vi "_FPGA_DDS_BMem_of_Cosine.vi"(8 "Addr":enum16{"Addr A", "Addr B"}(ring)=enum."Addr B", 10 "Cycle_in":u32, 11 "NormAmp*2^29":u32) -> (2 "cos":fxp<+/-,16,14>)   [LabVIEW 2018]
uses:
  <vilib>/rvi/Memory/Memory_Emulation/nirvimemoryFastEmulation.vi
  <vilib>/rvi/Memory/Memory_Emulation/nirvimemoryEmulation.vi
  <vilib>/rvi/Emulation/niFpgaEmulationIsFPGAContextNoSignature.vi
  <vilib>/rvi/DataTransferAndStorage/Container/Common/niFpgaContainerGetUniqueNameForEmu.vi
  <vilib>/rvi/Emulation/niFpgaProcessEmulError.vi
  <vilib>/rvi/Emulation/niFpgaSctlEmulationGetInTimedLoop.vi
  <vilib>/rvi/errors/nirviReportUnexpectedCaseInternalError (U32).vi
  <vilib>/rvi/DataTransferAndStorage/Container/XNode/niFpgaContainer.xnode
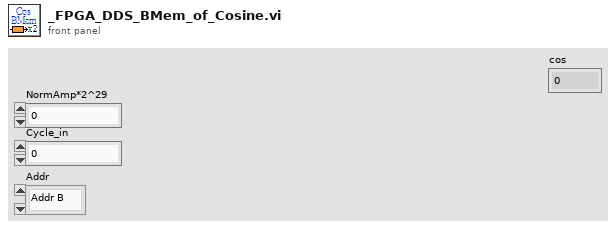
[diagram p1: front panel]
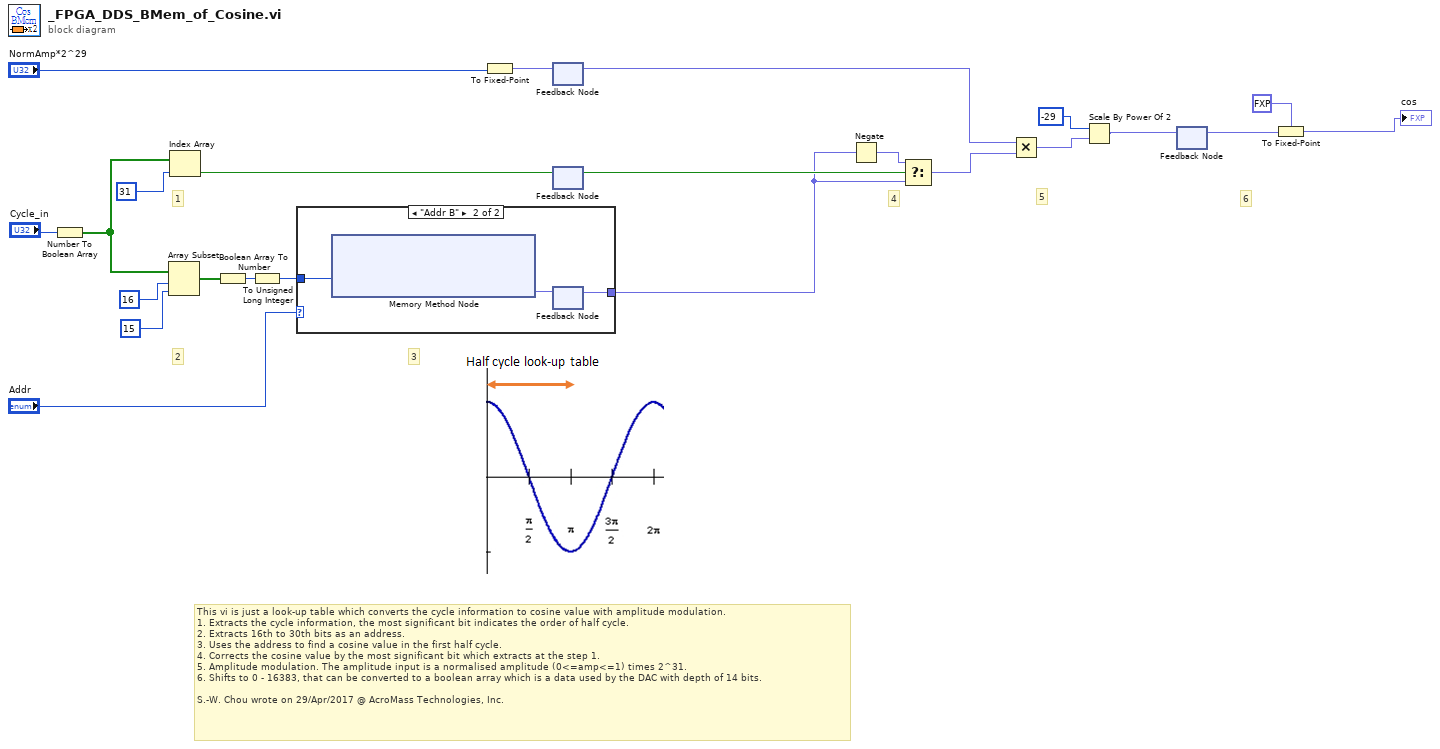
[diagram p0: block diagram]
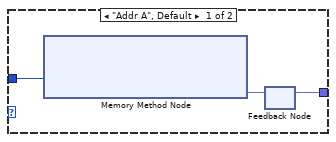
[diagram p2: hidden frame]
diagram:
  # "6"
  # "5"
  # "4"
  # "3"
  # "1"
  # "2"
  # "This vi is just a look-up table which converts the cycle information to cosine value with amplitude modulation.\n1. Extracts the cycle information, the most significant bit indicates the order of half cycle.\n2. Extracts 16th to 30th bits as an address.\n3. Uses the address to find a cosine value in the first half cycle.\n4. Corrects the cosine value by the most significant bit which extracts at the step 1.\n5. Amplitude modulation. The amplitude input is a normalised amplitude (0<=amp<=1) times 2^31.\n6. Shifts to 0 - 16383, that can be converted to a boolean array which is a data used by the DAC with depth of 14 bits.\n\nS.-W. Chou wrote on 29/Apr/2017 @ AcroMass Technologies, Inc."
  n1 = Number To Boolean Array(number="Cycle_in") -> (Boolean array=w21:bool[])
  n2 = Array Subset(array=w21, index=16, length=15 ("index")) -> (w19:bool[])
  n3 = Index Array(array=w21, index=31) -> (element=w5:bool)
  n4 = Boolean Array To Number(Boolean array=w19) -> (number=w18:u16)
  n5 = To Unsigned Long Integer(number=w18) -> (unsigned 32bit integer=w17:u32)
  n6 = case shown="\"Addr B\"" "Addr" {
    tunnel: w17 -> [w26 w29]
    tunnel: [w24 w27] -> w11
    frame "Addr A", Default {
      n7 = xnode ("Memory Method Node")("Address A"=w26) -> ("Data A"=w25:fxp<+/-,16,14>)  [unwired: 1 in, 1 out]
      n8 = feedback #1() -> (w24:fxp<+/-,16,14>)  [unwired: 1 in]
      n9 = feedback-in #1(w25) -> ()
    }
    frame "Addr B" {
      n10 = xnode ("Memory Method Node")("Address B"=w29) -> ("Data B"=w28:fxp<+/-,16,14>)  [unwired: 1 in, 1 out]
      n11 = feedback #2() -> (w27:fxp<+/-,16,14>)  [unwired: 1 in]
      n12 = feedback-in #2(w28) -> ()
    }
  }
  n13 = To Fixed-Point(number="NormAmp*2^29") -> (fixed-point=w10:fxp<+,32,32>)  [unwired: 1 in]
  n14 = feedback-in #3(w10) -> ()
  n15 = feedback #3() -> (w4:fxp<+,32,32>)  [unwired: 1 in]
  n16 = feedback-in #4(w5) -> ()
  n17 = feedback #4() -> (w16:bool)  [unwired: 1 in]
  n18 = Negate(x=w11) -> (-x=w12:fxp<+/-,17,15>)
  n19 = Select(t=w12, s=w16, f=w11) -> (s? t:f=w7:fxp<+/-,17,15>)
  n20 = Multiply(x=w4, y=w7) -> (x*y=w8:fxp<+/-,48,46>)
  n21 = Scale By Power Of 2(n=i16 -29, x=w8) -> (x*2^n=w6:fxp<+/-,48,46>)
  n22 = feedback #5() -> (w3:fxp<+/-,48,46>)  [unwired: 1 in]
  n23 = feedback-in #5(w6) -> ()
  n24 = To Fixed-Point(fixed-point type=fxp<+/-,16,14> 0.0 ("cos"), number=w3) -> (fixed-point=→"cos":fxp<+/-,16,14>)
